vi "6_VNA_const_GENERATOR_2Dsweep_power_frequency.vi"() -> ()   [LabVIEW 2013]
panel:
  out "Estimated time (minutes)":dbl=83.5 caption="Center Freq (Hz):" format="%#.6p"
  in  "?":enum32{"Generator"}(tab)
  in  "Freq_end (Hz)":dbl=20.0 caption="Center Freq (Hz):" min=1.0 max=20.0 format="%#.6p"
  in  "Freq_start (Hz)":dbl=2.0 caption="Center Freq (Hz):" min=1.0 max=19.0 format="%#.6p"
  in  "freq_points":i32=201
  in  "Power_start":dbl=-50.0 caption="Center Freq (Hz):" min=1.0 max=20.0 format="%#.6p"
  in  "Power_end":dbl caption="Center Freq (Hz):" min=1.0 max=19.0 format="%#.6p"
  in  "power_points":i32=20
  in  "?":enum32{"VNA"}(tab)
  in  "Automatic switch off?":bool=TRUE
  in  "?":enum32{"VNA"}(tab)
  in  "No averages":i32=4 caption="Center Freq (Hz):"
  in  "VNA power (dBm)":dbl=-10.0 caption="Center Freq (Hz):" format="%#.6p"
  in  "Center Freq (Hz)":dbl=2000000000.0 caption="Center Freq (Hz):" format="%#.6p"
  in  "Bandwidth (Hz)":dbl=10.0 caption="Center Freq (Hz):" format="%#.6p"
  out "Amplitude Raw":dbl[][](graph)
  out "VNA Reflceted Amplitude":dbl[](graph)=[0.058026663141328864, 0.05803849795427559, 0.05811703937725734, 0.05815581269373555, 0.05773074500489757, 0.057974056018262235, 0.05792263973344623, 0.05798436960826535, 0.05794488234507935, 0.05798570694063102, 0.05784771720783975, 0.05795338407956457, 0.057840843671274525, 0.058089918033549785, 0.058019092615871924, 0.05800064828925515, 0.057898786928891166, 0.05786872759374009, 0.0580100043741242, 0.05793470142149833, 0.058079830900258395, 0.05805122189456112, 0.058063558000027674, 0.05806857524034771, 0.05813040912188735, 0.05797159541667526, 0.05790926723035759, 0.05799707164655489, 0.058070768500696736, 0.05791171722460772, 0.057981247510288166, 0.05767221043354753, 0.057965661948100745, 0.05810030924436889, 0.057915998961230154, 0.05797566814836004, 0.05795786548302913, 0.05805369161784312, 0.05787893533271955, 0.05806673207858148, 0.058261978841988374, 0.057947725628452795, 0.05810902047894416, 0.05805648694696775, 0.05821758284529301, 0.058013828077984594, 0.058099596569018516, 0.05797751425266722, 0.05793490372338021, 0.05802061396290935, 0.057970352584750105, 0.05803229174103594, 0.0579637882534195, 0.0580350410270849, 0.058082929423698984, 0.05804382992438525, 0.05797717027726529, 0.05823822226118882, 0.05794508871587131, 0.05781285119756002, 0.05797336228713899, 0.05805552545355902, 0.0580493321766601, 0.05784120607160099, 0.058146657812212135, 0.05811707902931314, 0.05807561949473191, 0.05799692819311307, 0.05812585587814979, 0.05794758420666987, 0.05794519646147103, 0.057965686071082635, 0.05802565501386559, 0.058055118123842, 0.057923051256140064, 0.05815459074614384, 0.05809748564807492, 0.05802127503676257, 0.058085852498793805, 0.058180290029116066, 0.057965296913875225, 0.05793486974083068, 0.0580869733466499, 0.05798377501339084, 0.05790704162723868, 0.05794282475538721, 0.05810362373684792, 0.05805784052097211, 0.057938522485869254, 0.058076492264199496, 0.05808063722198564, 0.05810405068843348, 0.05801027127742878, 0.0579799839472041, 0.05813593253002459, 0.05807185184004468, 0.05793072589336637, 0.05808609650747513, 0.058029440438147395, 0.0578401607960717, 0.058123284776130046, 0.058173103979776375, 0.05817855551404137, 0.05805664938221305, 0.05815637577798108, 0.057955308265694144, 0.05806766550092498, 0.05794944123245471, 0.058082710542915736, 0.05819134746279538, 0.057741954621475924, 0.05822105766104357, 0.058061424675434424, 0.05796466936493169, 0.05800934349888875, 0.05820147862726091, 0.05810258499736625, 0.05822935152630262, 0.05798775946137623, 0.05784658399610158, 0.05784381050235382, 0.057829397089108905, 0.05802015081854871, 0.05803846083452325, 0.05792379624170108, 0.05795001926898748, 0.05833985802553164, 0.0580574450596022, 0.058103613907050024, 0.0579232543801039, 0.05801218614974536, 0.057955307714735484, 0.05809834911300535, 0.05801522733212914, 0.05787845150932581, 0.057901652471088035, 0.05797943837468677, 0.05802469293837562, 0.058011445067638216, 0.05809535088902378, 0.05797918748564069, 0.058188461726417, 0.0580395908875329, 0.05800473605839797, 0.0580688515835752, 0.058017568136421185, 0.057873972477131615, 0.05808662569904864, 0.05805413123624696, 0.058018499078984445, 0.05787344605223016, 0.058008557730744786, 0.05804306553419997, 0.05793390477108833, 0.057778690913912543, 0.058075912047088965, 0.057967245452416896, 0.05800538430473594, 0.057928166833695255, 0.05789988992389351, 0.05797333017682102, 0.057931774087793916, 0.05800626955719995, 0.057887372330670636, 0.058093759958342636, 0.05802334642727178, 0.05790022237014166, 0.05804715432434068, 0.05803332279732489, 0.057891628832557294, 0.0579804356513236, 0.05821470247415357, 0.0579514732246119, 0.058031950410890105, 0.058039807287309966, 0.05813819195778313, 0.0581223656270603, 0.058108681897048715, 0.0580453560517971, 0.05795663421609115, 0.058084596219921604, 0.05827744295243, 0.05810979680775561, 0.05780829172710737, 0.058023181472839414, 0.057896590713048826, 0.05788799523250717, 0.057896026872038465, 0.05798169843372059, 0.057920158898835936, 0.057686551444485104, 0.058000068137918956, 0.05814351596171303, 0.05806436466566891, 0.057915662986168216, 0.05812797515280926, 0.058158868330737995, 0.05809434936914437, 0.05807580219614148, 0.058069768703772166, 0.05802856979719687, 0.057927296055430816, 0.057785723827369156, 0.057983210153238755, 0.05819441199195606, 0.05809437545313067, 0.057922782429474025, 0.05815764398488769, 0.058060561341259045, 0.058101844690270875, 0.05805110866283839, 0.05788235828318604, 0.05794676783319845, 0.05807607890956949, 0.058003650765087136, 0.05794951848509215, 0.058011370346618935, 0.05808375066934293, 0.05791862147820358, 0.05806809978380321, 0.058029321990878596, 0.05801110708205415, 0.05823748023980829, 0.05800517974200871, 0.05805853349844117, 0.058087333322665975, 0.05788774235758308, 0.058060627534154884, 0.058194176461209085, 0.05790156238345011, 0.05792562167186391, 0.0579962971627144, 0.05806091756463454, 0.058052634589402755, 0.058020375028836856, 0.05816990977664673, 0.05795783030519389, 0.05791901147522786, 0.05811625136990784, 0.058256897629090004, 0.05810615871916794, 0.05800437961118808, 0.0578355695753206, 0.057977476765135476, 0.05804281379367141, 0.058006793894061576, 0.05780789083629374, 0.057781213483484826, 0.058073970079616316, 0.057808274775356897, 0.058210849821522616, 0.058057706347862566, 0.05810776023680018, 0.05790762223489207, 0.05796479363663274, 0.057941264375335026, 0.05793773738559963, 0.05829346411666525, 0.057994286340653095, 0.05802781162174649, 0.057913546015466104, 0.05787777153694701, 0.057958429090311764, 0.05791566195821273, 0.058065060747843567, 0.05774832061032806, 0.05820225401713783, 0.058097886704141545, 0.05806381030514724, 0.057918624894288846, 0.058095020571045604, 0.05808116494959369, 0.05787502033580458, 0.05808389901728728, 0.057978618845967805, 0.057989300555139234, 0.05809458208384878, 0.05803138920804645, 0.0578532593464961, 0.0580464643116841, 0.05801415425240238, 0.05782022145373558, 0.057950804496453595, 0.05789232855773969, 0.05782197013543651, 0.058046277452274544, 0.05808258564678685, 0.05801242752268905, 0.05824381838221222, 0.05776762564870695, 0.05779790259655375, 0.05817207642455946, 0.0581721746739324, 0.05799248435462356, 0.05799279007783535, 0.05769942530032417, 0.0580025232303214, 0.05798992463577151, 0.05789541601796913, 0.05805408471219325, 0.05801579144138166, 0.05786855049309419, 0.057964887877209416, 0.058161395957249395, 0.05815539081030705, 0.05803480900308704, 0.05784729813159695, 0.0579999989278052, 0.05796447118481649, 0.058020161547573605, 0.0580844110313773, 0.05794830656940934, 0.05814086407072948, 0.058072967721452505, 0.05791197718245686, 0.05794661991384289, 0.05816891284473762, 0.0580095723906255, 0.0580504164068092, 0.057960709079702986, 0.05778232061679917, 0.05784534699386978, 0.05785831511388573, 0.05807258521247955, 0.057990521135936175, 0.05791667605511446, 0.05793210154886452, 0.05798805957689641, 0.05803756540370877, 0.05786685442161563, 0.05794731453598156, 0.05788984175810983, 0.05816613545827039, 0.05798651969695663, 0.05785477154246905, 0.05821912066604688, 0.05810544783613655, 0.057991967561275226, 0.057766574669638346, 0.05812420298791922, 0.0581821180337577, 0.05801606889717017, 0.058073672856977204, 0.058019174498308575, 0.05800904460457746, 0.05790491707146801, 0.05817475004857513, 0.05792014953364437, 0.05795842460285771, 0.05790870628431516, 0.058122798646086646, 0.0579549621371007, 0.058068681165643045, 0.057904478418788256, 0.05776808329532924, 0.05770594741312335, 0.058023470296405845, 0.05812131922527412, 0.05799212315696688, 0.05804702892682736, 0.057832119464226374, 0.05791737689425913, 0.05807578806130643, 0.05793403413625629, 0.05788278335895478, 0.05792708105644899, 0.05815607433046263, 0.057912849460022855, 0.05808356728241779, 0.05805894899086111, 0.058013679504095965, 0.05824107142402651, 0.05792559753555554, 0.057877002751882664, 0.058112680668026134, 0.05805256265615851, 0.057924191681894166, 0.05799479472865945, 0.05788263133758165, 0.0579508231782606, 0.05815500188870022, 0.057839560031765366, 0.057818175058956416, 0.057890931672544076, 0.05816639849760669, 0.057879429842116754, 0.057944673882589066, 0.05801485768864072, 0.05789087802873832, 0.05767117180365048, 0.058054998154953505, 0.057975244869268985, 0.057798191053235304, 0.058170296810765625, 0.058031568559273106, 0.057984076944176524, 0.057961228221831786, 0.05792747437702453, 0.05794991395164056, 0.05804557472936662, 0.05779279186425183, 0.057941539753710414, 0.05793638312657315, 0.05784932476131088, 0.05808007509124251, 0.057889852743626645, 0.05791676422418222, 0.0579633339070995, 0.05800509193072238, 0.0579944879402366, 0.05789156147186153, 0.05823233238266043, 0.05808470981687092, 0.058030580498876196, 0.05784740270841621, 0.05787380478247587, 0.05810072940314053, 0.05799439030690191, 0.057710126651123794, 0.05807343009586362, 0.0580156766634388, 0.058039033613119136, 0.05831148448176001, 0.05783181043421043, 0.057935916811891704, 0.05809594900231087, 0.05795005323695443, 0.05783241776757722, 0.05792810109920746, 0.05789433950850385, 0.05791938091682445, 0.058105438117713085, 0.05791344926020419, 0.05796862414024386, 0.05801358480956299, 0.05817649505966406, 0.057782135420096206, 0.05794165669700932, 0.0580524154400223, 0.057764559798325926, 0.05811436460966107, 0.05824103686050407, 0.05801053654976288, 0.058091163733072604, 0.058085358523335545, 0.05802901711959458, 0.05805360684040213, 0.058062465455238785, 0.05786469679857622, 0.058043660475349784, 0.05782077467040617, 0.05823379884193517, 0.058027186497825664, 0.05781844577280796, 0.05796197015690267, 0.05812982556094596, 0.05809832871833364, 0.058179335216101094, 0.05795537700363129, 0.057916507699201134, 0.05805118231458261, 0.05796648865111608, 0.05801192080445169, 0.057843241447421645, 0.0579148248644517, 0.057957318100457095, 0.05785103885018981, 0.057954005272576374, 0.058161247459376696, 0.05808848179153845, 0.05795029202167759, 0.05809891590918398, 0.05797719621088747, 0.057806667932484755, 0.057964527848030856, 0.057912692893044, 0.0580778231883156, 0.05813755331031676, 0.058039071203879584, 0.05808923773587676, 0.058044812859864646, 0.05788766976236418, 0.05798770039429804, 0.05799174063803184, 0.05798772934723883, 0.057944658180251456, 0.058125694161047965, 0.058065564757984744, 0.05801658301868459, 0.05792629880497905, 0.058071631862724446, 0.05792720143691027, 0.057941566225668435, 0.05796087934358523, 0.057965899109209455, 0.05810962355517424, 0.05812043393203238, 0.05799884068472175, 0.057914413026840326, 0.057789371956235853, 0.05790278121696356]
  out "VNA Reflceted Phase":dbl[](graph)=[-2.131909511286724, -2.127049291071839, -2.1298315868870303, -2.1311558363355703, -2.1291457409964623, -2.1314268958401272, -2.1322816240821143, -2.128458862186085, -2.132762465209358, -2.132293699882456, -2.1285648264874264, -2.1311689241645295, -2.1310314665976997, -2.131055387854716, -2.1293807804938534, -2.1276022427141807, -2.1333667986620712, -2.129188413998661, -2.130591912764168, -2.130788479262257, -2.1288860750093024, -2.1284707825198383, -2.129402375249564, -2.128454651073532, -2.1308823309228986, -2.1262095206384846, -2.1262847792348327, -2.128760815354333, -2.1281550814798487, -2.1264071215832714, -2.126295744457205, -2.127438914939761, -2.128305675467529, -2.1334606650741073, -2.130793875212272, -2.1312496116592863, -2.128202600439076, -2.1316899127489153, -2.12789340903039, -2.125564435294478, -2.126234062177974, -2.126732495287123, -2.127096108408488, -2.129265832561903, -2.1303623634337003, -2.1303805621750236, -2.1285496256628393, -2.130199403389061, -2.1290315200087058, -2.127340373314344, -2.129486932547821, -2.1288738222407977, -2.1301835782666796, -2.1313680100395755, -2.131919073029006, -2.131417204700565, -2.1319092536781468, -2.129348442664714, -2.1312735798978193, -2.132183127595387, -2.1312599332648516, -2.1318468731865123, -2.1309649064631127, -2.1324554772247097, -2.1279200817029524, -2.1310779792557355, -2.1365176901568272, -2.131583707063495, -2.1343963426992727, -2.132570340519514, -2.1339162778922063, -2.128900076851594, -2.1328158663298704, -2.133209424572771, -2.1291268710088413, -2.1298958798990384, -2.1295689579072232, -2.128401030626821, -2.1292813656048266, -2.133800221727447, -2.129881057598837, -2.129518091551091, -2.130679438419548, -2.1291871490734424, -2.1270640395740057, -2.126245982361593, -2.131208908775766, -2.1297059711585806, -2.1278740037690307, -2.1289122916155727, -2.1285520534753912, -2.1272904022184354, -2.127248697878283, -2.1299082263288858, -2.127904045673292, -2.1320611496007507, -2.128727347303898, -2.12758999836544, -2.1285616297240275, -2.126825485529375, -2.1325621310530893, -2.128065588629912, -2.127804797319367, -2.12772933662971, -2.1291993640533375, -2.1293081388861523, -2.1297504234992144, -2.12972969785636, -2.129885387952614, -2.1317187247782137, -2.131439554642937, -2.1292044055184642, -2.1269690064386664, -2.128644373778767, -2.1335213778788433, -2.1330267161755847, -2.1329279603763713, -2.1304355663399805, -2.132457405691605, -2.13287370463415, -2.1349194120746104, -2.1289084592286733, -2.1291808302478406, -2.130987506156394, -2.1311361707297927, -2.1325814882070775, -2.129070307059719, -2.128657701856902, -2.1306409521455008, -2.1282076798390555, -2.1295408616293967, -2.129841189161127, -2.1310263744738998, -2.1307309598527424, -2.1316048635180773, -2.1303938730174083, -2.1310068776343964, -2.128083766953352, -2.1272684948440093, -2.127993000679656, -2.129492286350107, -2.1273508334693907, -2.128854192434158, -2.1269083525872134, -2.1310927227594822, -2.1287676892892327, -2.125617054632976, -2.128857771795623, -2.12712568973459, -2.1292119487174683, -2.1285681710692694, -2.1272212494529503, -2.1282394518048138, -2.127168068807711, -2.12680729401357, -2.127369144005565, -2.1252308000374356, -2.128016276479212, -2.128007141873094, -2.1275367714664735, -2.1305062087828834, -2.1304779480502742, -2.1292260771102502, -2.1277820169706905, -2.1290636034631163, -2.1285146564256396, -2.1311381277398307, -2.1292396479576943, -2.126958759048806, -2.131079801601639, -2.128385513422585, -2.1299522873660983, -2.1315814242920763, -2.1294784736518246, -2.1335041864606668, -2.1318475712362868, -2.131467025285111, -2.131427209183751, -2.1366359419345704, -2.1309863889923473, -2.1318243179281473, -2.1288167280792636, -2.129785684332419, -2.1321707457331143, -2.1292889246187077, -2.1299416914204263, -2.1295510371551782, -2.131862213824649, -2.13442495071802, -2.1313363767151987, -2.132424520470009, -2.1304745440111605, -2.134109070514616, -2.131358939892051, -2.130756259238289, -2.1292819512204613, -2.129142927482591, -2.127574676034729, -2.129923524102218, -2.129442369344591, -2.1285425646039524, -2.1323801130912328, -2.1325955656987774, -2.1284309536260806, -2.133020071611059, -2.1304459545079872, -2.1286103317465956, -2.1295852402150692, -2.129937612725993, -2.1311157526297286, -2.1277522972157548, -2.1305197883011253, -2.129137992925284, -2.1330007464703673, -2.125409778148802, -2.1269874983927304, -2.1281727268833155, -2.1274636534677995, -2.1304997300834088, -2.1279701828490616, -2.129507173931959, -2.1292397507951404, -2.1268415574944615, -2.1276726728199984, -2.1294239900168384, -2.13068254331922, -2.132164704375514, -2.129422927848508, -2.129378204624776, -2.1295556802817064, -2.1305929655651448, -2.1339027204782215, -2.1299636888185414, -2.1306331973566395, -2.1304068936479803, -2.1312335022786395, -2.1291603447339056, -2.1312682458514582, -2.1312258473038703, -2.1309200480517494, -2.1325457298199635, -2.1309493293010653, -2.131686503060326, -2.129136070559979, -2.1292951997579355, -2.131610645604282, -2.1324431960319634, -2.131357670594327, -2.1281567865032325, -2.1337127673832397, -2.127986591482452, -2.1294880320492737, -2.131764729639308, -2.1314148186797497, -2.129701324084455, -2.12926593547654, -2.128393303799097, -2.1281928735795015, -2.1257553321514067, -2.1331496491422337, -2.128541597284467, -2.1305403741076883, -2.1287668280558236, -2.1287285972092787, -2.129632291288226, -2.1259462336137576, -2.1309169585965977, -2.130844758177817, -2.128674910680314, -2.1289458083980874, -2.1282140071818074, -2.1281431535756123, -2.1322911819764485, -2.12942643025912, -2.1297488653523393, -2.126842982267688, -2.130142568251179, -2.1298513192157724, -2.1288954464363274, -2.1241095443298708, -2.1277488941095735, -2.1301332398321704, -2.126681949907033, -2.1331057248440914, -2.131395932405157, -2.134048764801784, -2.1315163924717946, -2.133824583511216, -2.1316383157306307, -2.131871730381053, -2.1288387699325444, -2.1323536906304823, -2.1264770557580195, -2.130617908630831, -2.132938467927775, -2.1293450227120205, -2.1317262935770565, -2.1335104586865765, -2.131568176496448, -2.1338859622746726, -2.1305894242774404, -2.133313602397618, -2.1283251801428578, -2.126249326296589, -2.132494897258511, -2.128752213137251, -2.1298695982861364, -2.1305796094087532, -2.1315843933341907, -2.132407751410363, -2.1292017354881163, -2.1292728095677567, -2.127125300807519, -2.1297614817605117, -2.12816349935943, -2.130365684641971, -2.1293800260713316, -2.131127953844377, -2.127429724203051, -2.129469068200722, -2.128129176123826, -2.128827331132275, -2.1298847648509596, -2.1256996031079347, -2.1286380873159008, -2.127622651982593, -2.127076593937206, -2.126159412881594, -2.127264618890454, -2.1290697353456207, -2.126607636462366, -2.1286980232852835, -2.130710047514779, -2.1270977101117, -2.1292668641253294, -2.125730772371237, -2.129546464069831, -2.1288994689815564, -2.1297587209650795, -2.1310698146831144, -2.1294907027824475, -2.128370052682691, -2.130289596935971, -2.1322094502723514, -2.13246554596718, -2.1285569232768022, -2.1285823611728913, -2.134614569440099, -2.134174159667569, -2.130540242895795, -2.127918917660741, -2.1317556973804836, -2.133446390621932, -2.1333499175425077, -2.123803865484325, -2.1321813963716894, -2.132310036680094, -2.1352032052534575, -2.130073884487657, -2.133289843829986, -2.1298733374702774, -2.1350590457000083, -2.133469308151594, -2.1287943620538017, -2.1284156291528853, -2.1277216975301787, -2.1294822979810157, -2.1308569709792304, -2.133927901603799, -2.1300513831887833, -2.131456347615896, -2.1289298892563586, -2.128613754953843, -2.1301617593037743, -2.1298668740118045, -2.1289406753519424, -2.127629032790045, -2.126340906604137, -2.1320801006253545, -2.13230209750835, -2.1307596435042058, -2.1295948138685104, -2.1272919709534936, -2.127412743409446, -2.125534850528987, -2.1289717261628027, -2.123932751297983, -2.127174440652112, -2.1262488016326557, -2.1262532073318696, -2.1283663084838746, -2.129307889245009, -2.127155263415932, -2.128605845915697, -2.1297272915720873, -2.1290842592295864, -2.130127282749878, -2.129337593003136, -2.1281681300855104, -2.1282310228952923, -2.13345050061961, -2.1329241980479847, -2.133930230677171, -2.1312747816321314, -2.135826462880827, -2.129268062926261, -2.1305435464295073, -2.1318329796742956, -2.134526483611433, -2.130162105757427, -2.1342425912173435, -2.1338849927645267, -2.1338835766973028, -2.1315802437347022, -2.131942924814701, -2.1310514672415817, -2.132445019724868, -2.1288812531052765, -2.1310691761922365, -2.1280542947073213, -2.1264849813504445, -2.131888611165528, -2.1332366969814442, -2.132909124252242, -2.1309847578475827, -2.1318853044296695, -2.129917413768197, -2.128653126109212, -2.1338478359122566, -2.130380533167807, -2.1328452508980353, -2.129381757303441, -2.128337234933103, -2.127798996949861, -2.1302975700949873, -2.130887825792639, -2.127001569203819, -2.1308333468925245, -2.131550362087834, -2.1293529813296828, -2.127150872291021, -2.1292531544951574, -2.1303360252117454, -2.126584329274897, -2.1288283510543424, -2.129413724678454, -2.1264510128588485, -2.129938481218499, -2.127086408681894, -2.1275751502945264, -2.1292423947479278, -2.1292639099986648, -2.1297756553300142, -2.129136100025875, -2.130760207471152, -2.1274203121621578, -2.1308619903734103, -2.1348871438672306, -2.1301391770924525, -2.12836543777363, -2.1309188689751806, -2.1305559360078004, -2.1299071563550966, -2.1332406354981037, -2.1315509255807603, -2.129034567276479, -2.1333933799027074, -2.1327136045405415, -2.1328243692634743, -2.1303817784657597, -2.1349648652950277, -2.131821821457068, -2.130012860779474, -2.1316546025270755, -2.1316177146925, -2.1338792419538746, -2.129913586848288, -2.130714322136911, -2.131058898367296, -2.1307500229558474, -2.129599475525236, -2.133192356838146, -2.13336901368948, -2.131785195676379, -2.136010508941394, -2.128778909023022, -2.129384624690344, -2.1304440191441314, -2.12784778762697, -2.1307536275652312, -2.128425134693412, -2.1276403761106852, -2.1286190908788747, -2.1269214220055033, -2.129951810237312, -2.131182902633483, -2.1296939964752464, -2.128862824743932, -2.1304407477583425, -2.1276290917496876, -2.130641045999957]
  out "Phase  Corrected":dbl[][](graph)
  out "Amplitude Corrected":dbl[][](graph)
  out "Phase Raw":dbl[][](graph)
  # "dBm"
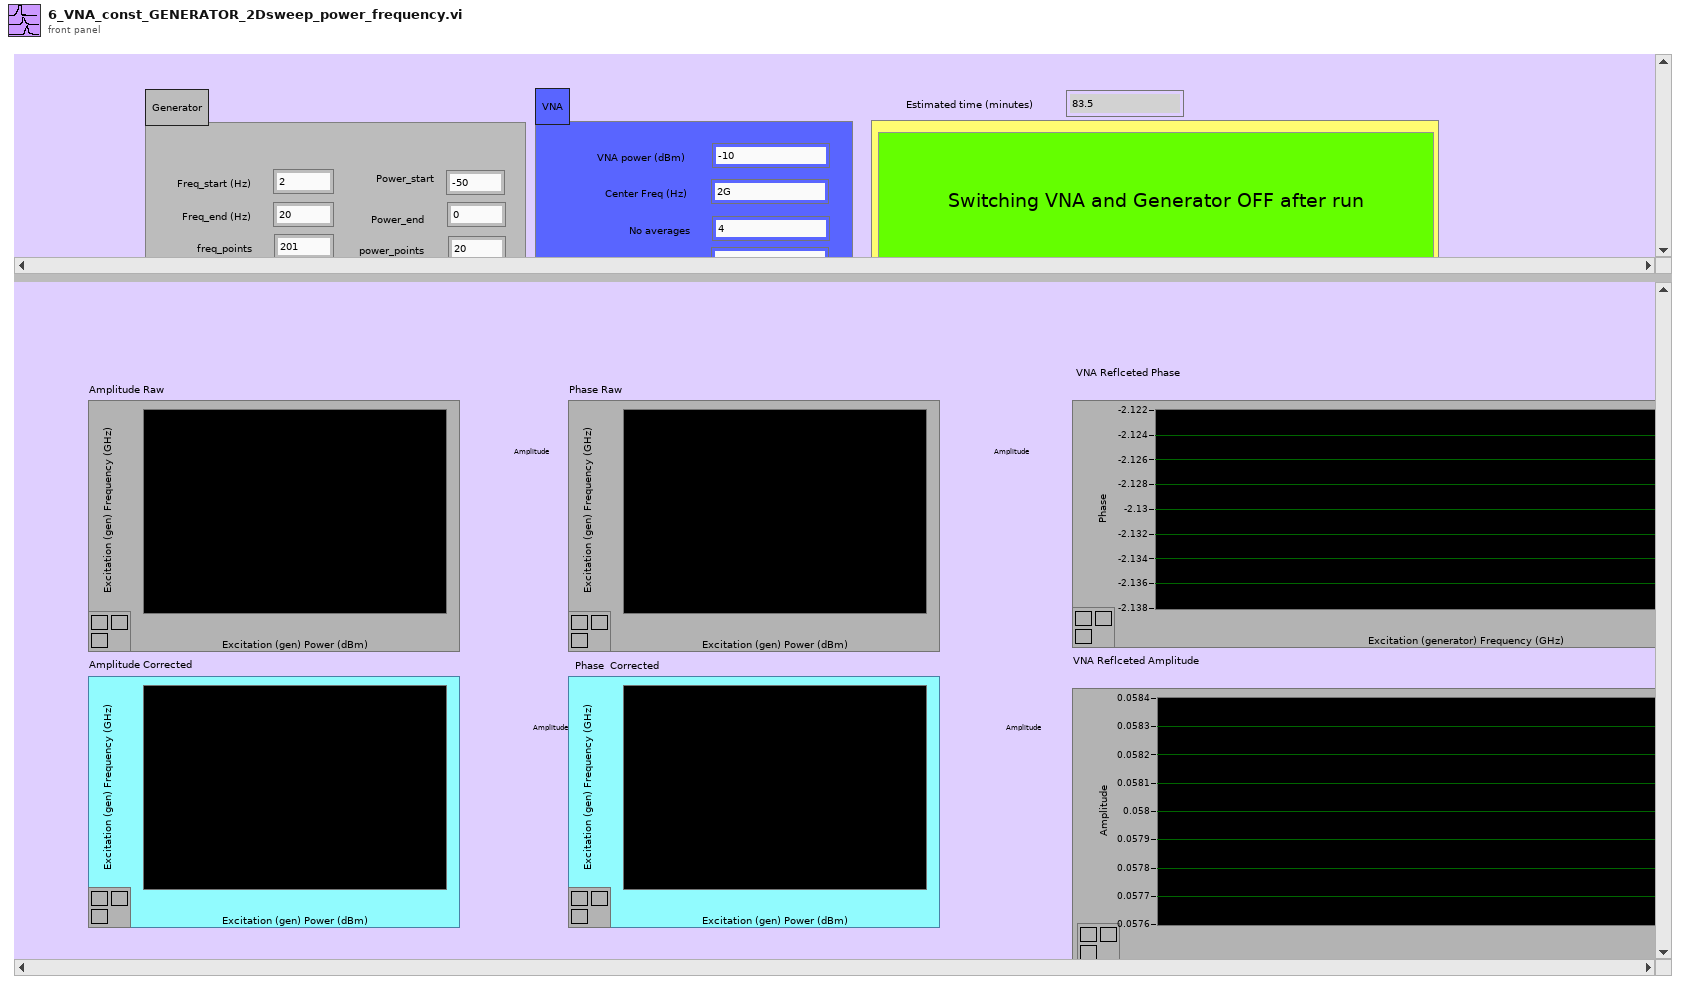
[diagram p1: front panel]
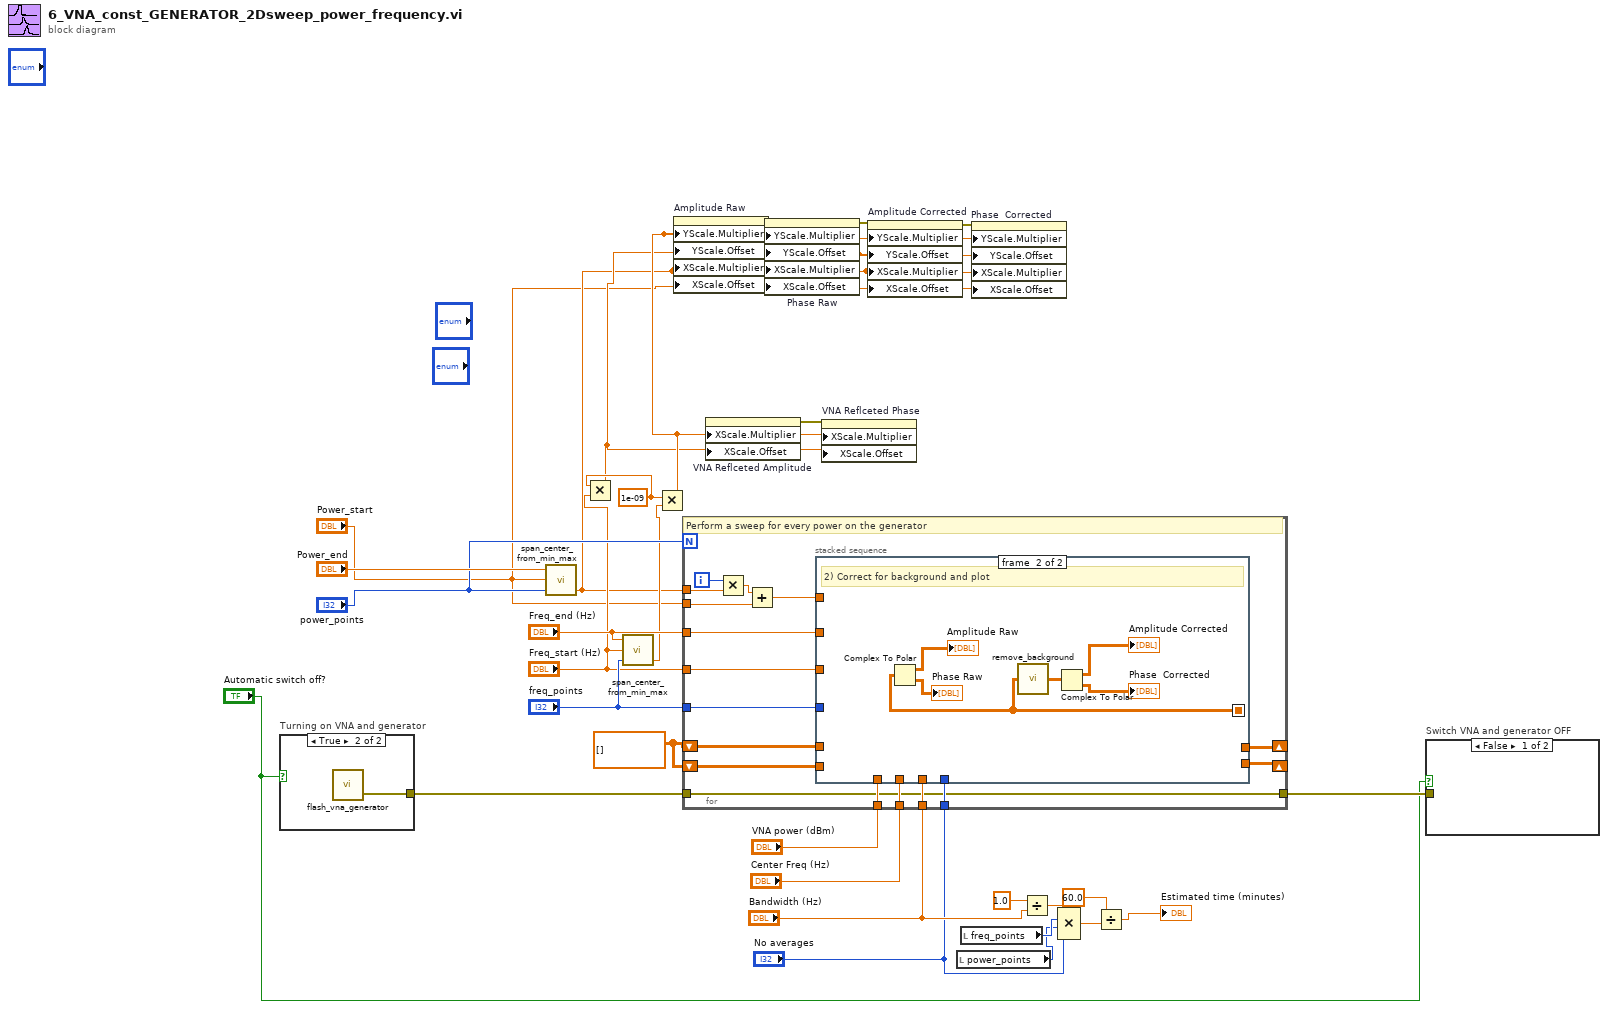
[diagram p0: block diagram]
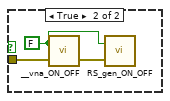
[diagram p2: hidden frame]
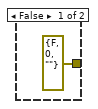
[diagram p3: hidden frame]
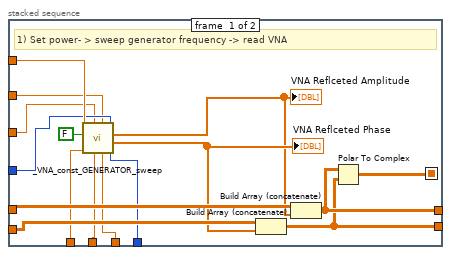
[diagram p4: hidden frame]
diagram:
  w6 = 1e-09 ("x")
  w27 = dbl[][] []
  n1 = case "Turning on VNA and generator" shown="True" "Automatic switch off?" {
    tunnel: [errorcluster {"status"=FALSE, "code"=0, "source"=""} ("error out") w32] -> w20
    frame False {
    }
    frame True {
      n2 = call "flash_vna_generator.vi"() -> ("error out"=w32:errorcluster)  [unwired: 3 in]
    }
  }
  n3 = call "span_center_from_min_max.vi"("No Points"="power_points", "Begin"="Power_start", "End"="Power_end") -> ("Step"=w2:dbl)  [unwired: 2 out]
  n4 = Multiply(x=w6, y="Freq_start (Hz)") -> (x*y=w3:dbl)
  n5 = call "span_center_from_min_max.vi"("No Points"="freq_points", "Begin"="Freq_start (Hz)", "End"="Freq_end (Hz)") -> ("Step"=w8:dbl)  [unwired: 2 out]
  n6 = Multiply(x=w6, y=w8) -> (x*y=w4:dbl)
  n7 = property on="Amplitude Raw" class="IntGraph (strict)"("YScale.Multiplier"=w4, "YScale.Offset"=w3, "XScale.Multiplier"=w2, "XScale.Offset"="Power_start") -> (error out=w5:errorcluster)  [unwired: 2 in, 1 out]
  n8 = for {
    N: "power_points" -> [_]
    shift-right: [w35] -> _
    shift-left: w27 -> [w37]
    tunnel: "Power_start" -> [w46]
    tunnel: w2 -> [w48]
    tunnel: "Freq_end (Hz)" -> [w45]
    tunnel: "Freq_start (Hz)" -> [w44]
    tunnel: "freq_points" -> [w43]
    tunnel: "VNA power (dBm)" -> [w41]
    tunnel: "Center Freq (Hz)" -> [w40]
    tunnel: "Bandwidth (Hz)" -> [w39]
    tunnel: "No averages" -> [w38]
    shift-right: [w34] -> _
    shift-left: w27 -> [w36]
    tunnel: w20 -> [w33]
    tunnel: [w33] -> w19
    i -> [w49]
    # "Perform a sweep for every power on the generator"
    n9 = Multiply(x=w49, y=w48) -> (x*y=w47:dbl)
    n10 = Add(x=w47, y=w46) -> (x+y=w42:dbl)
    n11 = stacked-sequence {
      seq-local: [w63 _] -> [_ w71]
      tunnel: w45 -> [w56 _]
      tunnel: w44 -> [w57 _]
      tunnel: w43 -> [w59 _]
      tunnel: w42 -> [w60 _]
      tunnel: w41 -> [w55 _]
      tunnel: w40 -> [w54 _]
      tunnel: w39 -> [w53 _]
      tunnel: w38 -> [w52 _]
      tunnel: w37 -> [w64 _]
      tunnel: w36 -> [w65 _]
      tunnel: [w62 _] -> w35
      tunnel: [w61 _] -> w34
      frame #0 {
        # "1) Set power- > sweep generator frequency -> read VNA"
        n12 = call "_VNA_const_GENERATOR_sweep.vi"("VNA power (dBm)"=w55, "Center Freq (Hz)"=w54, "Bandwidth (Hz)"=w53, "No averages"=w52, "Turn off VNA and generator?"=FALSE, "Gen power (dBm)"=w60, "Freq_start (Hz)"=w57, "Freq_end (Hz)"=w56, "n_points"=w59) -> ("VNA Reflected Phase"=w51:dbl[], "VNA Reflected Amplitude"=w50:dbl[])  [unwired: 1 in]
        "VNA Reflceted Amplitude" <- w50
        "VNA Reflceted Phase" <- w51
        n13 = Build Array (concatenate)(w65, w51) -> (w61:dbl[][])
        n14 = Build Array (concatenate)(w64, w50) -> (w62:dbl[][])
        n15 = Polar To Complex(1:w61, 2:w62) -> (0:w63:cdb[][])
      }
      frame #1 {
        # "2) Correct for background and plot"
        n16 = Complex To Polar(r * e^(i*theta)=w71) -> (r=→"Amplitude Raw":dbl[][], theta=→"Phase Raw":dbl[][])
        n17 = call "remove_background.vi"("Array in"=w71) -> ("Array out"=w69:cdb[][])  [unwired: 1 in]
        n18 = Complex To Polar(r * e^(i*theta)=w69) -> (r=→"Amplitude Corrected":dbl[][], theta=→"Phase  Corrected":dbl[][])
      }
    }
  }
  n19 = property on="VNA Reflceted Amplitude" class="WFGraph (strict)"("XScale.Multiplier"=w4, "XScale.Offset"=w3) -> (error out=w21:errorcluster)  [unwired: 2 in, 1 out]
  n20 = property on="Phase Raw" class="IntGraph (strict)"(error in=w5, "YScale.Multiplier"=w4, "YScale.Offset"=w3, "XScale.Multiplier"=w2, "XScale.Offset"="Power_start") -> (error out=w24:errorcluster)  [unwired: 1 in, 1 out]
  n21 = property on="VNA Reflceted Phase" class="WFGraph (strict)"(error in=w21, "XScale.Multiplier"=w4, "XScale.Offset"=w3) -> ()  [unwired: 1 in, 2 out]
  n22 = property on="Amplitude Corrected" class="IntGraph (strict)"(error in=w24, "YScale.Multiplier"=w4, "YScale.Offset"=w3, "XScale.Multiplier"=w2, "XScale.Offset"="Power_start") -> (error out=w25:errorcluster)  [unwired: 1 in, 1 out]
  n23 = local read "power_points"() -> (w10:i32)
  n24 = local read "freq_points"() -> (w11:i32)
  n25 = property on="Phase  Corrected" class="IntGraph (strict)"(error in=w25, "YScale.Multiplier"=w4, "YScale.Offset"=w3, "XScale.Multiplier"=w2, "XScale.Offset"="Power_start") -> ()  [unwired: 1 in, 2 out]
  n26 = Divide(x=1.0, y="Bandwidth (Hz)") -> (x/y=w16:dbl)
  n27 = Compound Arithmetic op=MULTIPLY(w16, w11, w10, "No averages") -> (w15:dbl)
  n28 = Divide(x=w15, y=60.0) -> (x/y=→"Estimated time (minutes)":dbl)
  n29 = case "Switch VNA and generator OFF" shown="False" "Automatic switch off?" {
    tunnel: w19 -> [_ w72]
    frame False {
    }
    frame True {
      w73 = FALSE ("VNA Output")
      n30 = call "__vna_ON_OFF.vi"("VNA Output"=w73, "error in (no error)"=w72) -> ("error out"=w74:errorcluster)
      n31 = call "RS_gen_ON_OFF.vi"("Generator Output"=w73, "error in (no error)"=w74) -> ()  [unwired: 1 out]
    }
  }
